vi "UpdateWFGraphScaleColorAsPlotColor.vi"(7 "Plots#":i32=4, 8 "error in (no error)":errorcluster, 11 "WaveformGraph in":refnum<vi>) -> (0 "error out":errorcluster)   [LabVIEW 2020]
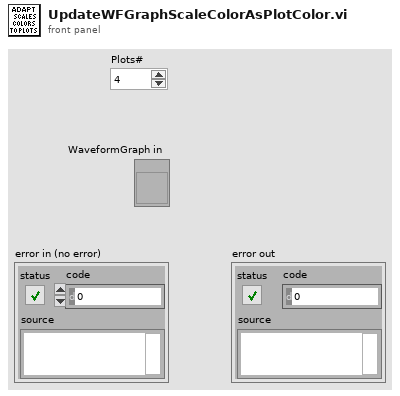
[diagram p1: front panel]
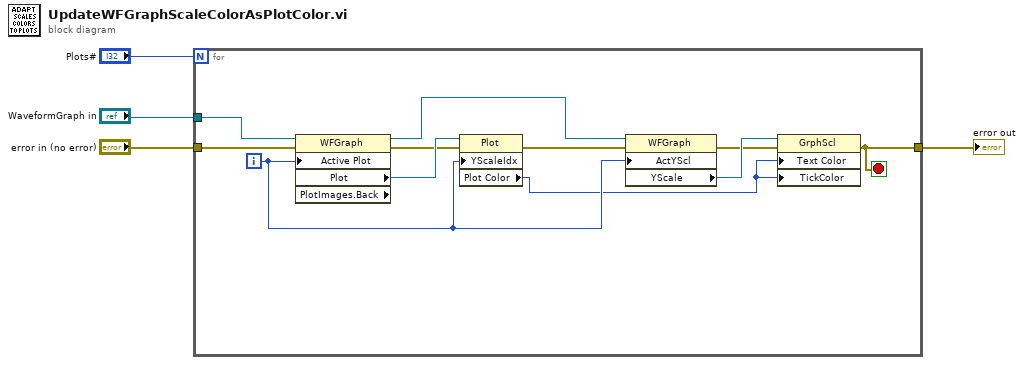
[diagram p0: block diagram]
diagram:
  n1 = for {
    N: "Plots#" -> [_]
    tunnel: "WaveformGraph in" -> [w15]
    tunnel: "error in (no error)" -> [w11]
    tunnel: [w5] -> w4
    i -> [w8]
    stop <- w5 stop-if-true
    n2 = property class="WFGraph" props=["Active Plot", "Plot", "PlotImages.Back"](reference=w15, error in=w11, "Active Plot"=w8) -> (reference out=w9:refnum<vi>, error out=w10:errorcluster, "Plot"=w14:refnum<vi>)  [unwired: 1 out]
    n3 = property class="Plot"(reference=w14, error in=w10, "YScaleIdx"=w8) -> (error out=w13:errorcluster, "Plot Color"=w6:u32)  [unwired: 1 out]
    n4 = property class="WFGraph"(reference=w9, error in=w13, "ActYScl"=w8) -> (error out=w7:errorcluster, "YScale"=w12:refnum<vi>)  [unwired: 1 out]
    n5 = property class="GrphScl"(reference=w12, error in=w7, "Text Color"=w6, "TickColor"=w6) -> (error out=w5:errorcluster)  [unwired: 1 out]
  }
  "error out" <- w4
